vi "Get Bucket Versioning.vi"(8 "error in (no error)":errorcluster, 11 "Bucket in":refnum<class "Bucket.lvclass">) -> (0 "error out":errorcluster, 1 "MFA Delete":T1, 2 "Status":T2, 3 "Bucket out":refnum<class "Bucket.lvclass">)   [LabVIEW 2015, in "NI_AWS_S3.lvlib" / "Bucket.lvclass"]
doc: "This implementation of the GET operation uses the versioning subresource to return the versioning state of a bucket. To retrieve the versioning state of a bucket, you must be the bucket owner."
uses:
  Bucket.lvclass
  Versioning Status.ctl
  MFA Delete.ctl
  Core/HTTP Request/Region handling.ctl
  Core/HTTP Request/Request Options.ctl
  Core/HTTP Request/Name Value Pair.ctl
  Core/HTTP Request/URL formatting.ctl
  Bucket.lvclass/Bucket.ctl
  Read Name.vi
  Core/HTTP Request/HTTP Request.lvclass
  XML Parsing/NI_XML Parsing.lvlib
  NI_AWS_S3.lvlib
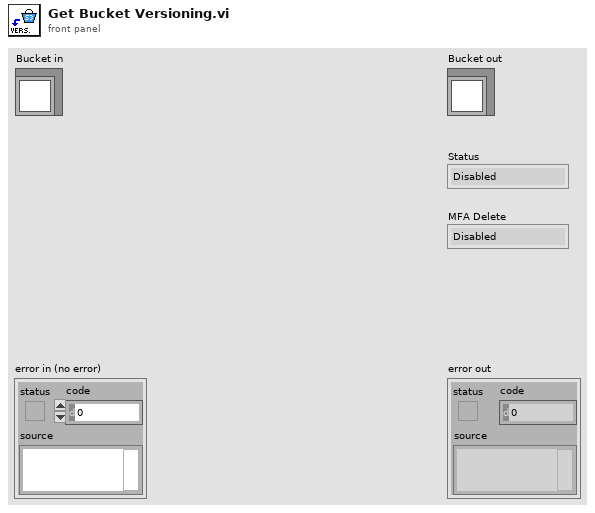
[diagram p1: front panel]
types:
  T1 = typedef "NI_AWS_S3.lvlib/MFA Delete.ctl" = enum16{"Disabled", "Enabled"}
  T2 = typedef "NI_AWS_S3.lvlib/Versioning Status.ctl" = enum16{"Disabled", "Suspended", "Enabled"}
  T3 = typedef "NI_AWS_Core.lvlib/HTTP Request.lvclass/Name Value Pair.ctl" = cluster{"name":string, "value":string}
  T4 = typedef "NI_AWS_Core.lvlib/HTTP Request.lvclass/Request Options.ctl" = cluster{"request headers":T3[], "request parameters":T3[], "request body":string, "region handling":T5, "URL formatting":T6}
  T5 = typedef "NI_AWS_Core.lvlib/HTTP Request.lvclass/Region handling.ctl" = enum16{"use region everywhere", "use region (authentication only)", "use region (URL only)", "ignore region everwhere"}
  T6 = typedef "NI_AWS_Core.lvlib/HTTP Request.lvclass/URL formatting.ctl" = enum16{"region-", "region."}
  T7 = typedef "NI_AWS_Core.lvlib/HTTP Request.lvclass/Response.ctl" = cluster{"Headers":string, "Body":string}
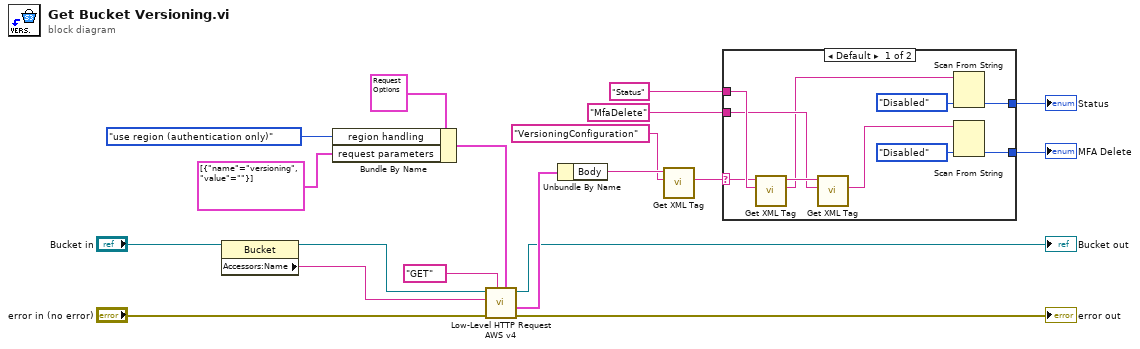
[diagram p0: block diagram]
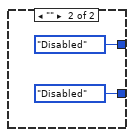
[diagram p2: hidden frame]
diagram:
  n1 = property class="Bucket"(reference="Bucket in") -> (reference out=w2:refnum<class "Bucket.lvclass">, "Accessors:Name"=w19:string)  [unwired: 1 in, 1 out]
  n2 = Bundle By Name(cluster=T4 {"request headers"=[], "request parameters"=[], "request body"="", "region handling"=enum."use region everywhere", "URL formatting"=enum."region."} ("Request Options"), "region handling"=Region_handling."use region (authentication only)", "request parameters"=T3[] [{"name"="versioning", "value"=""}]) -> (w3:T4)
  n3 = call "Low-Level HTTP Request AWS v4.vi"("Request Options"=w3, "HTTP-Verb"="GET", "error in (no error)"="error in (no error)", "URL Prefix"=w19, "AWS Core in"=w2) -> ("error out"=→"error out":errorcluster, "Response"=w5:T7, "AWS Core out"=→"Bucket out":refnum<class "Bucket.lvclass">)  [unwired: 3 in, 1 out]
  n4 = Unbundle By Name(w5) -> ("Body"=w12:string)
  n5 = call "Get XML Tag.vi"("Tag name"="VersioningConfiguration", "XML String in"=w12) -> ("Tag value"=w10:string)  [unwired: 5 in, 4 out]
  n6 = case shown="Default" w10 {
    selector: w10 -> [w20 _]
    tunnel: [w22 Versioning_Status."Disabled" ("Status")] -> w9
    tunnel: [w23 MFA_Delete."Disabled" ("MFA Delete")] -> w8
    tunnel: "Status" ("Tag name") -> [w29 _]
    tunnel: "MfaDelete" ("Tag name") -> [w27 _]
    frame Default {
      n7 = call "Get XML Tag.vi"("Tag name"=w29, "XML String in"=w20) -> ("Tag value"=w26:string, "XML String dup"=w28:string)  [unwired: 5 in, 3 out]
      n8 = call "Get XML Tag.vi"("Tag name"=w27, "XML String in"=w28) -> ("Tag value"=w21:string)  [unwired: 5 in, 4 out]
      n9 = Scan From String(input string=w26, default 1=Versioning_Status."Disabled" ("Status")) -> (output 1=w22:T2)  [unwired: 3 in, 3 out]
      n10 = Scan From String(input string=w21, default 1=MFA_Delete."Disabled" ("MFA Delete")) -> (output 1=w23:T1)  [unwired: 3 in, 3 out]
    }
    frame "" {
    }
  }
  "Status" <- w9
  "MFA Delete" <- w8
